vi "deleteProductDataInProductTable.vi"(8 "error in":errorcluster, 11 "dataReadingToDelete":T1) -> (0 "error out":errorcluster)   [LabVIEW 2014]
uses:
  <vilib>/addons/database/Connection.llb/DB Tools Open Connec (String).vi
  <vilib>/addons/database/NI_Database_API.lvlib
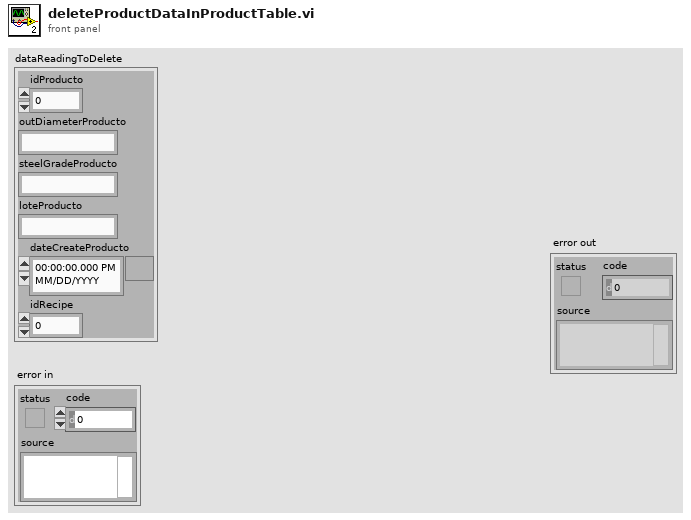
[diagram p1: front panel]
types:
  T1 = cluster{"idProducto":dbl, "outDiameterProducto":string, "steelGradeProducto":string, "loteProducto":string, "dateCreateProducto":timestamp, "idRecipe":dbl}
  T2 = typedef "NI_Database_API.lvlib/Conn ObjectReference.ctl" = refnum<k1>
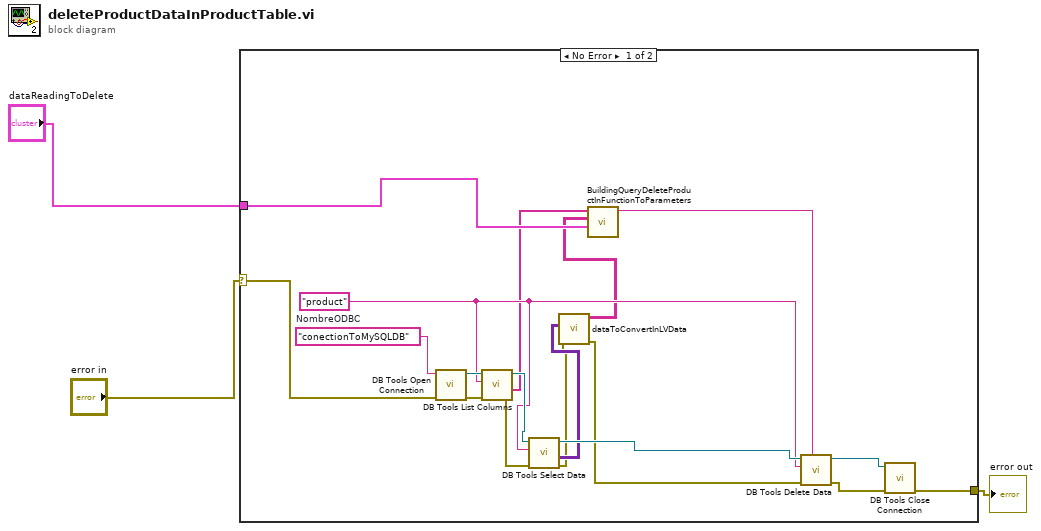
[diagram p0: block diagram]
diagram:
  n1 = case shown="No Error" "error in" {
    selector: "error in" -> [w8 w22]
    tunnel: "dataReadingToDelete" -> [w7 _]
    tunnel: [w9 w22] -> w3
    frame No Error {
      w16 = "product" ("table")
      w21 = "conectionToMySQLDB"  # NombreODBC
      n2 = call-poly <vilib>:"DB Tools Open Connection.vi"("error in (no error)"=w8, "connection information"=w21) -> ("error out"=w19:errorcluster, "connection reference"=w20:T2)  [unwired: 6 in]
      n3 = call <vilib>:"DB Tools List Columns.vi"("error in (no error)"=w19, "table"=w16, "connection reference"=w20) -> ("error out"=w15:errorcluster, "columns"=w5:string[], "connection reference out"=w18:T2)  [unwired: 1 in, 1 out]
      n4 = call <vilib>:"DB Tools Select Data.vi"("error in (no error)"=w15, "table"=w16, "connection reference"=w18) -> ("error out"=w13:errorcluster, "data"=w14:variant[][], "connection reference out"=w17:T2)  [unwired: 3 in]
      n5 = call "dataToConvertInLVData.vi"("error in"=w13, "dataReadingIn"=w14) -> ("error out"=w12:errorcluster, "dataReadingOut"=w6:string[][])  [unwired: 8 in]
      n6 = call "BuildingQueryDeleteProductInFunctionToParameters.vi"("dataReadingToDelete"=w7, "dataReadingOut"=w6, "columns"=w5) -> ("queryToDelete"=w4:string)  [unwired: 8 in]
      n7 = call <vilib>:"DB Tools Delete Data.vi"("condition"=w4, "error in (no error)"=w12, "table"=w16, "connection reference"=w17) -> ("error out"=w10:errorcluster, "connection reference out"=w11:T2)  [unwired: 6 in]
      n8 = call <vilib>:"DB Tools Close Connection.vi"("error in (no error)"=w10, "connection reference"=w11) -> ("error out"=w9:errorcluster)  [unwired: 5 in]
    }
    frame Error {
    }
  }
  "error out" <- w3
